vi "FeedForward.vi"(6 "a1":dbl, 7 "a2":dbl, 9 "x1_norm":dbl, 10 "x1_ref_norm_dot":dbl, 11 "x2":dbl) -> (3 "TFF":dbl)   [LabVIEW 2013]
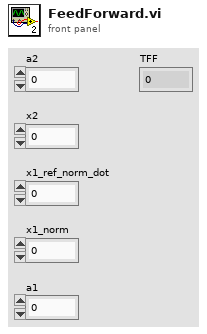
[diagram p1: front panel]
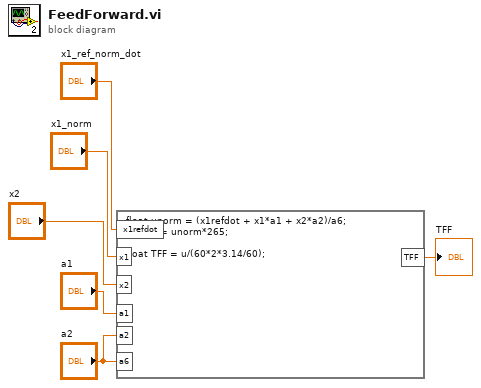
[diagram p0: block diagram]
diagram:
  n1 = formula code="float unorm = (x1refdot + x1*a1 + x2*a2)/a6;\nfloat u = unorm*265;\n\nfloat TFF = u/(60*2*3.14/60);"("x1refdot"="x1_ref_norm_dot", "x1"="x1_norm", "x2"="x2", "a2"="a2", "a1"="a1", "a6"="a2") -> ("TFF"=→"TFF":dbl)
